vi "PH_4_Pos_Selector.Picture MA MM1 Bend.vi"(1 "State":T1 items=["unknown", "Position I", "Position II", "Position III", "Position IV", "moving"]) -> (0 "Array MM1 Bend":picture[](array[picture]))   [LabVIEW 2014, in "PH_4_Pos_Selector.lvlib"]
uses:
  PH_4_Pos_Selector.lvlib
  PH_4_Pos_Selector.Position Selector.ctl
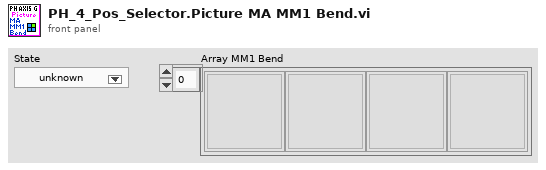
[diagram p1: front panel]
types:
  T1 = typedef "PH_4_Pos_Selector.lvlib/PH_4_Pos_Selector.Position Selector.ctl" = u16
  T2 = cluster{"Font Name:":string, "Size":i16, "Strikeout?":bool, "Italic?":bool, "Underline?":bool, "Outline?":bool, "Shadow?":bool, "Bold?":bool}
  T3 = cluster{"left":i16, "top":i16, "right":i16, "bottom":i16}[]
  T4 = cluster{"left":i16, "top":i16, "right":i16, "bottom":i16}
  T5 = cluster{"horizontal":enum16{"left", "center", "right"}, "vertical":enum16{"top", "center", "bottom"}}
  T6 = cluster{"Width":u16, "Style":enum32{"Solid", "Dash", "Dot", "DashDot", "DashDotDot"}}
  T7 = enum16{"User-specified Font", "Application Font", "System Font", "Dialog Font"}
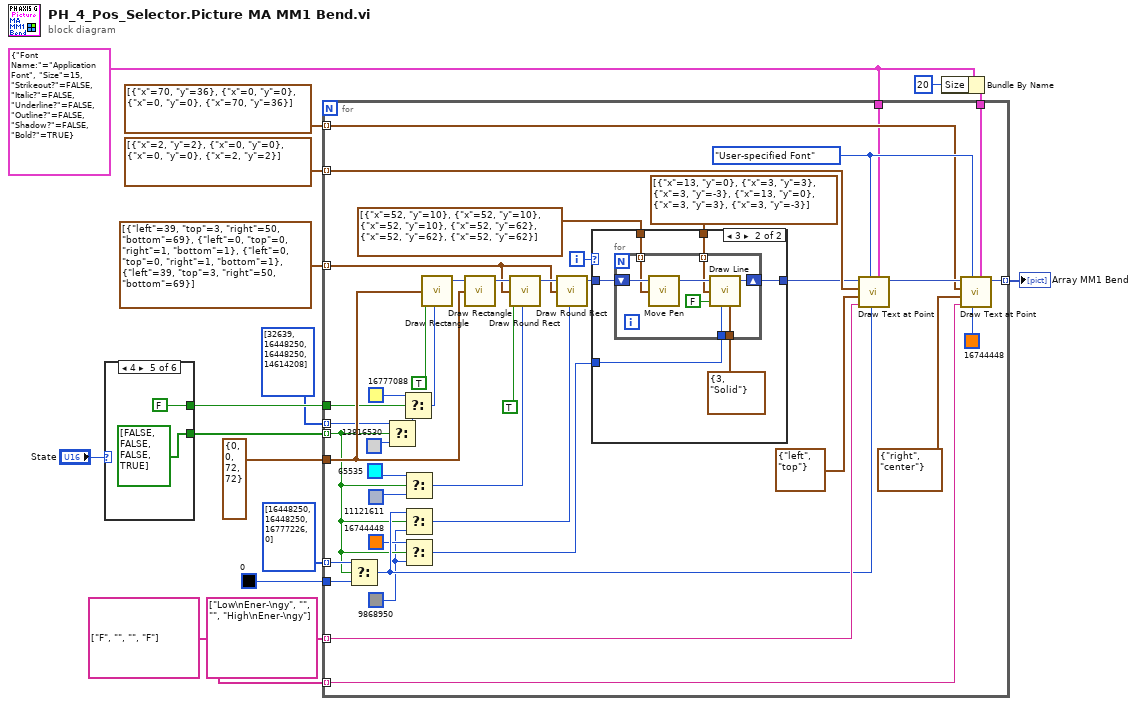
[diagram p0: block diagram]
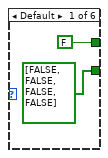
[diagram p2: hidden frame]
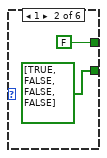
[diagram p3: hidden frame]
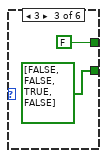
[diagram p4: hidden frame]
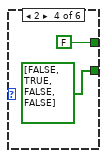
[diagram p5: hidden frame]
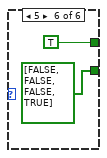
[diagram p6: hidden frame]
diagram:
  w2 = T2 {"Font Name:"="Application Font", "Size"=15, "Strikeout?"=FALSE, "Italic?"=FALSE, "Underline?"=FALSE, "Outline?"=FALSE, "Shadow?"=FALSE, "Bold?"=TRUE} ("[user-specified font]")
  n1 = case shown="4" "State" {
    tunnel: [bool[] [FALSE, FALSE, FALSE, FALSE] bool[] [TRUE, FALSE, FALSE, FALSE] bool[] [FALSE, FALSE, TRUE, FALSE] bool[] [FALSE, TRUE, FALSE, FALSE] bool[] [FALSE, FALSE, FALSE, TRUE] bool[] [FALSE, FALSE, FALSE, TRUE]] -> w14
    tunnel: [FALSE FALSE FALSE FALSE FALSE TRUE] -> w13
    frame Default {
    }
    frame 1 {
    }
    frame 3 {
    }
    frame 2 {
    }
    frame 4 {
    }
    frame 5 {
    }
  }
  n2 = Bundle By Name(cluster=w2, "Size"=i16 20) -> (w3:T2)
  n3 = for {
    tunnel: T4 {"left"=0, "top"=0, "right"=72, "bottom"=72} ("rect") -> [w68]
    tunnel: w14 -> [w45] mode=indexing
    tunnel: w13 -> [w65]
    tunnel: [w37] -> w16 mode=indexing
    tunnel: string[] ["Low\nEner-\ngy", "", "", "High\nEner-\ngy"] -> [w61] mode=indexing
    tunnel: u32[] [32639, 16448250, 16448250, 14614208] -> [w60] mode=indexing
    tunnel: u32[] [16448250, 16448250, 16777226, 0] -> [w59] mode=indexing
    tunnel: u32 0 -> [w58]
    tunnel: cluster{"x":i16, "y":i16}[] [{"x"=2, "y"=2}, {"x"=0, "y"=0}, {"x"=0, "y"=0}, {"x"=2, "y"=2}] -> [w49] mode=indexing
    tunnel: T3 [{"left"=39, "top"=3, "right"=50, "bottom"=69}, {"left"=0, "top"=0, "right"=1, "bottom"=1}, {"left"=0, "top"=0, "right"=1, "bottom"=1}, {"left"=39, "top"=3, "right"=50, "bottom"=69}] -> [w50] mode=indexing
    tunnel: string[] ["F", "", "", "F"] -> [w35] mode=indexing
    tunnel: cluster{"x":i16, "y":i16}[] [{"x"=70, "y"=36}, {"x"=0, "y"=0}, {"x"=0, "y"=0}, {"x"=70, "y"=36}] -> [w32] mode=indexing
    tunnel: w2 -> [w30]
    tunnel: w3 -> [w29]
    i -> [w41]
    w44 = u32 9868950
    w34 = T7."User-specified Font" ("desired font(Application)")
    n4 = Select(t=w59, s=w45, f=w58) -> (s? t:f=w52:u32)
    n5 = Select(t=w60, s=w45, f=u32 13816530) -> (s? t:f=w63:u32)
    n6 = Select(t=u32 16777088, s=w65, f=w63) -> (s? t:f=w62:u32)
    n7 = Select(t=u32 65535 ("color(black)"), s=w45, f=u32 11121611) -> (s? t:f=w54:u32)
    n8 = Select(t=w52, s=w45, f=w44) -> (s? t:f=w51:u32)
    n9 = Select(t=u32 16744448 ("color(black)"), s=w45, f=w44) -> (s? t:f=w43:u32)
    n10 = call <vilib>:"Draw Rectangle.vi"("rect"=w68, "fill?(F)"=TRUE, "color(black)"=w62) -> ("new picture"=w69:picture)  [unwired: 6 in]
    n11 = call <vilib>:"Draw Rectangle.vi"("picture"=w69, "rect"=w68) -> ("new picture"=w57:picture)  [unwired: 7 in]
    n12 = call <vilib>:"Draw Round Rect.vi"("picture"=w57, "rect"=w50, "fill?(F)"=TRUE, "color(black)"=w54) -> ("new picture"=w56:picture)  [unwired: 5 in]
    n13 = call <vilib>:"Draw Round Rect.vi"("picture"=w56, "rect"=w50, "color(black)"=w51) -> ("new picture"=w42:picture)  [unwired: 6 in]
    n14 = case shown="3" w41 {
      tunnel: [w70 w76] -> w47
      tunnel: w43 -> [_ w75]
      tunnel: w42 -> [w70 w73]
      tunnel: cluster{"x":i16, "y":i16}[] [{"x"=52, "y"=10}, {"x"=52, "y"=10}, {"x"=52, "y"=10}, {"x"=52, "y"=62}, {"x"=52, "y"=62}, {"x"=52, "y"=62}] -> [_ w72]
      tunnel: cluster{"x":i16, "y":i16}[] [{"x"=13, "y"=0}, {"x"=3, "y"=3}, {"x"=3, "y"=-3}, {"x"=13, "y"=0}, {"x"=3, "y"=3}, {"x"=3, "y"=-3}] -> [_ w71]
      frame Default {
      }
      frame 3 {
        n15 = for {
          tunnel: w75 -> [w83]
          tunnel: T6 {"Width"=3, "Style"=enum."Solid"} ("pen") -> [w82]
          tunnel: w72 -> [w78] mode=indexing
          shift-right: [w84] -> w76
          shift-left: w73 -> [w81]
          tunnel: w71 -> [w77] mode=indexing
          n16 = call <vilib>:"Move Pen.vi"("new position"=w78, "picture"=w81) -> ("new picture"=w80:picture)  [unwired: 3 in]
          n17 = call <vilib>:"Draw Line.vi"("picture"=w80, "end point"=w77, "absolute coordinates?(T)"=FALSE, "color(black)"=w83, "pen"=w82) -> ("new picture"=w84:picture)  [unwired: 4 in]
        }
      }
    }
    n18 = call <vilib>:"Draw Text at Point.vi"("[user-specified font]"=w30, "text color(black)"=w52, "desired font(Application)"=w34, "text"=w61, "alignment(left, top)"=T5 {"horizontal"=enum."left", "vertical"=enum."top"}, "origin"=w49, "picture"=w47) -> ("new picture"=w38:picture)  [unwired: 3 in, 1 out]
    n19 = call <vilib>:"Draw Text at Point.vi"("[user-specified font]"=w29, "text color(black)"=u32 16744448 ("color(black)"), "desired font(Application)"=w34, "text"=w35, "alignment(left, top)"=T5 {"horizontal"=enum."right", "vertical"=enum."center"}, "origin"=w32, "picture"=w38) -> ("new picture"=w37:picture)  [unwired: 3 in, 1 out]
  }
  "Array MM1 Bend" <- w16
